vi "XLP80_HH_Basic.vi"(7 "Function":string, 8 "err in":errorcluster) -> (0 "err out":errorcluster)   [LabVIEW 2021]
doc: "This example demonstrates a basic configuration and measurement task with an electronic load."
uses:
  XLP80_HH_TDefsCluster_HH Feedback.ctl
  XLP80_HH_TDefsCluster_HH Setpoint.ctl
  XLP80_HH_Globals.vi
  XLP80_General_Libs/HH_Libs/HH PLI Series.lvlib
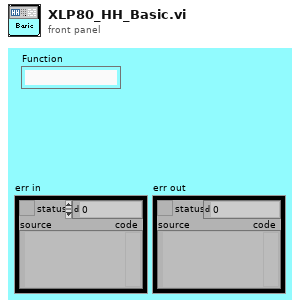
[diagram p1: front panel]
types:
  T1 = typedef "XLP80_HH_TDefsCluster_HH Setpoint.ctl" = cluster{"Enable Input":bool, "Set Current":sgl, "Set Voltage":sgl, "Set Power":sgl}
  T2 = cluster{"Baud Rate":u32, "Parity":u16, "Data Bits":u16, "Stop Bits":u16}
  T3 = typedef "XLP80_HH_TDefsCluster_HH Feedback.ctl" = cluster{"Current":sgl, "Voltage":sgl, "Power":sgl}
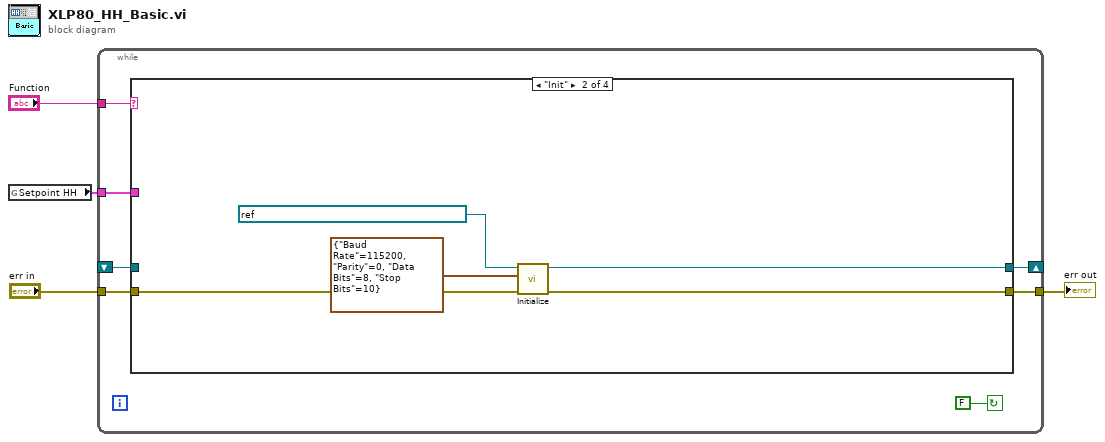
[diagram p0: block diagram]
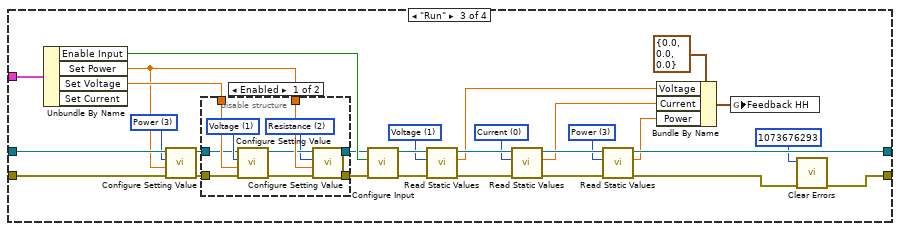
[diagram p3: hidden frame]
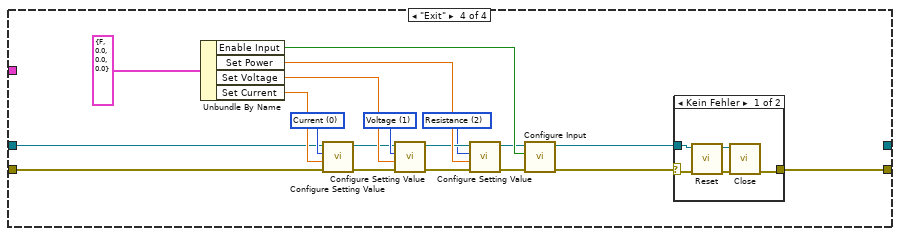
[diagram p5: hidden frame]
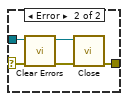
[diagram p6: hidden frame]
diagram:
  n1 = global read "XLP80_HH_Globals.vi" "Setpoint HH"() -> (w1:T1)
  n2 = while {
    tunnel: [w8] -> w2
    tunnel: "Function" -> [w7]
    shift-right: [w11] -> _
    shift-left: _ -> [w10]
    tunnel: "err in" -> [w6]
    tunnel: w1 -> [w5]
    stop <- FALSE continue-if-true
    n3 = case shown="\"Init\"" w7 {
      tunnel: [w13 w17 w42 _] -> w11
      tunnel: w10 -> [w13 _ w40 w63]
      tunnel: [w12 w18 w37 w78] -> w8
      tunnel: w6 -> [w12 w15 w36 w62]
      tunnel: w5 -> [_ _ w29 _]
      frame Default {
      }
      frame "Init" {
        n4 = call "Initialize.vi"("error in (no error)"=w15, "Serial Configuration"=T2 {"Baud Rate"=115200, "Parity"=0, "Data Bits"=8, "Stop Bits"=10}, "VISA resource name"=refnum<visa-resource-name> "TCPIP::192.168.150.100::1001::SOCKET") -> ("error out"=w18:errorcluster, "VISA resource name out"=w17:refnum<visa-resource-name>)  [unwired: 7 in]
      }
      frame "Run" {
        w20 = u16 3 items=["Current", "Voltage", "Resistance", "Power"] ("Operation Mode (0: Current)")
        w23 = u16 3 items=["Current", "Voltage", "Resistance", "Power", "Temperature", "MPPT Energy"] ("Measurement (0: Current)")
        w25 = u16 0 items=["Current", "Voltage", "Resistance", "Power", "Temperature", "MPPT Energy"] ("Measurement (0: Current)")
        w26 = u16 1 items=["Current", "Voltage", "Resistance", "Power", "Temperature", "MPPT Energy"] ("Measurement (0: Current)")
        n5 = Unbundle By Name(w29) -> ("Enable Input"=w32:bool, "Set Power"=w19:sgl, "Set Voltage"=w35:sgl)  [unwired: 1 out]
        n6 = call "Configure Setting Value.vi"("error in (no error)"=w36, "Setting Value (0)"=w19, "Operation Mode (0: Current)"=w20, "VISA resource name"=w40) -> ("error out"=w33:errorcluster, "VISA resource name out"=w34:refnum<visa-resource-name>)  [unwired: 6 in]
        n7 = disable-structure shown="Enabled" {
          disable-tunnel: w35 -> [w56 _]
          disable-tunnel: w34 -> [w55 w59]
          disable-tunnel: w33 -> [w54 w58]
          disable-tunnel: w19 -> [w53 _]
          disable-tunnel: [w50 w58] -> w31
          disable-tunnel: [w49 w59] -> w30
          frame Enabled {
            w48 = u16 2 items=["Current", "Voltage", "Resistance"] ("Operation Mode (0: Current)")
            w57 = u16 1 items=["Current", "Voltage", "Resistance"] ("Operation Mode (0: Current)")
            n8 = call "Configure Setting Value.vi"("error in (no error)"=w54, "Setting Value (0)"=w56, "Operation Mode (0: Current)"=w57, "VISA resource name"=w55) -> ("error out"=w51:errorcluster, "VISA resource name out"=w52:refnum<visa-resource-name>)  [unwired: 6 in]
            n9 = call "Configure Setting Value.vi"("error in (no error)"=w51, "Setting Value (0)"=w53, "Operation Mode (0: Current)"=w48, "VISA resource name"=w52) -> ("error out"=w50:errorcluster, "VISA resource name out"=w49:refnum<visa-resource-name>)  [unwired: 6 in]
          }
          frame Disabled {
          }
        }
        n10 = call "Configure Input.vi"("error in (no error)"=w31, "Enable Input State (False)"=w32, "VISA resource name"=w30) -> ("error out"=w46:errorcluster, "VISA resource name out"=w45:refnum<visa-resource-name>)  [unwired: 7 in]
        n11 = call "Read Static Values.vi"("error in (no error)"=w46, "Measurement (0: Current)"=w26, "VISA resource name"=w45) -> ("error out"=w47:errorcluster, "Measurement"=w27:dbl, "VISA resource name out"=w44:refnum<visa-resource-name>)  [unwired: 6 in]
        n12 = call "Read Static Values.vi"("error in (no error)"=w47, "Measurement (0: Current)"=w25, "VISA resource name"=w44) -> ("error out"=w41:errorcluster, "Measurement"=w24:dbl, "VISA resource name out"=w43:refnum<visa-resource-name>)  [unwired: 6 in]
        n13 = call "Read Static Values.vi"("error in (no error)"=w41, "Measurement (0: Current)"=w23, "VISA resource name"=w43) -> ("error out"=w38:errorcluster, "Measurement"=w22:dbl, "VISA resource name out"=w42:refnum<visa-resource-name>)  [unwired: 6 in]
        n14 = Bundle By Name(cluster=T3 {"Current"=0.0, "Voltage"=0.0, "Power"=0.0} ("Feedback HH"), "Voltage"=w27, "Current"=w24, "Power"=w22) -> (w21:T3)
        n15 = global write "XLP80_HH_Globals.vi" "Feedback HH"(w21) -> ()
        n16 = call <vilib>:"Clear Errors.vi"("error in (no error)"=w38, "specific error code to clear (0: all)"=1073676293) -> ("error out"=w37:errorcluster)  [unwired: 4 in, 1 out]
      }
      frame "Exit" {
        w65 = u16 2 items=["Current", "Voltage", "Resistance"] ("Operation Mode (0: Current)")
        w75 = u16 1 items=["Current", "Voltage", "Resistance"] ("Operation Mode (0: Current)")
        w77 = u16 0 items=["Current", "Voltage", "Resistance"] ("Operation Mode (0: Current)")
        n17 = Unbundle By Name(T1 {"Enable Input"=FALSE, "Set Current"=0.0, "Set Voltage"=0.0, "Set Power"=0.0} ("Setpoint HH")) -> ("Enable Input"=w68:bool, "Set Power"=w71:sgl, "Set Voltage"=w74:sgl, "Set Current"=w76:sgl)
        n18 = call "Configure Setting Value.vi"("error in (no error)"=w62, "Setting Value (0)"=w76, "Operation Mode (0: Current)"=w77, "VISA resource name"=w63) -> ("error out"=w72:errorcluster, "VISA resource name out"=w73:refnum<visa-resource-name>)  [unwired: 6 in]
        n19 = call "Configure Setting Value.vi"("error in (no error)"=w72, "Setting Value (0)"=w74, "Operation Mode (0: Current)"=w75, "VISA resource name"=w73) -> ("error out"=w69:errorcluster, "VISA resource name out"=w70:refnum<visa-resource-name>)  [unwired: 6 in]
        n20 = call "Configure Setting Value.vi"("error in (no error)"=w69, "Setting Value (0)"=w71, "Operation Mode (0: Current)"=w65, "VISA resource name"=w70) -> ("error out"=w67:errorcluster, "VISA resource name out"=w66:refnum<visa-resource-name>)  [unwired: 6 in]
        n21 = call "Configure Input.vi"("error in (no error)"=w67, "Enable Input State (False)"=w68, "VISA resource name"=w66) -> ("error out"=w60:errorcluster, "VISA resource name out"=w61:refnum<visa-resource-name>)  [unwired: 7 in]
        n22 = case shown="Kein Fehler" w60 {
          selector: w60 -> [w80 w84]
          tunnel: [w81 w87] -> w78
          tunnel: w61 -> [w79 w85]
          frame No Error {
            n23 = call "Reset.vi"("error in (no error)"=w80, "VISA resource name"=w79) -> ("error out"=w83:errorcluster, "VISA resource name out"=w82:refnum<visa-resource-name>)  [unwired: 8 in]
            n24 = call "Close.vi"("error in (no error)"=w83, "VISA resource name"=w82) -> ("error out"=w81:errorcluster)  [unwired: 9 in]
          }
          frame Error {
            n25 = call <vilib>:"Clear Errors.vi"("error in (no error)"=w84) -> ("error out"=w86:errorcluster)  [unwired: 5 in, 1 out]
            n26 = call "Close.vi"("error in (no error)"=w86, "VISA resource name"=w85) -> ("error out"=w87:errorcluster)  [unwired: 9 in]
          }
        }
      }
    }
  }
  "err out" <- w2
